vi "Write SPI.vi"(8 "error in (no error)":errorcluster, 10 "LINX SPI":refnum<class "LINX SPI.lvclass">, 11 "LINX-ADS1015 in":refnum<class "LINX-ADS1256.lvclass">) -> (0 "error out":errorcluster, 3 "LINX-ADS1015 out":refnum<class "LINX-ADS1256.lvclass">)   [LabVIEW 2020, in "LINX-ADS1256.lvclass"]
uses:
  LINX-ADS1256.lvclass
  LINX SPI/LINX SPI.lvclass
  LINX-ADS1256.lvclass/LINX-ADS1256.ctl
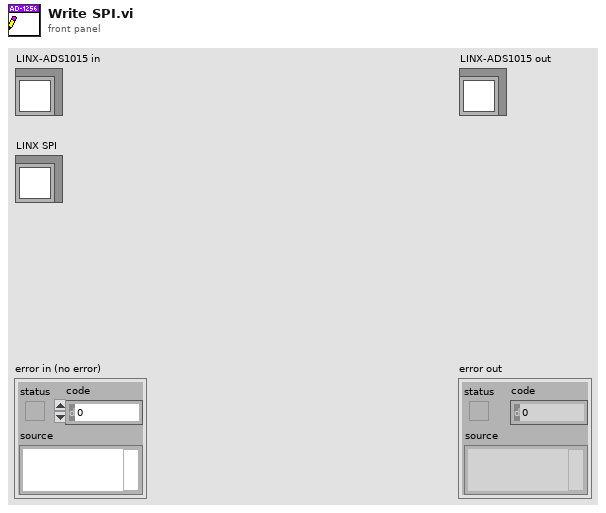
[diagram p1: front panel]
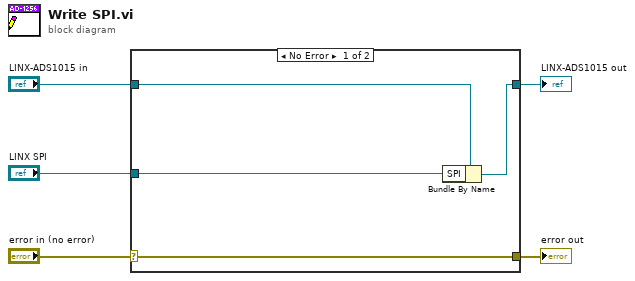
[diagram p0: block diagram]
diagram:
  n1 = case shown="No Error" "error in (no error)" {
    selector: "error in (no error)" -> [w9 w10]
    tunnel: [w9 w10] -> w4
    tunnel: [w7 w11] -> w2
    tunnel: "LINX-ADS1015 in" -> [w8 w11]
    tunnel: "LINX SPI" -> [w6 _]
    frame No Error {
      n2 = Bundle By Name(cluster=w8, "SPI"=w6) -> (w7:refnum<class "LINX-ADS1256.lvclass">)
    }
    frame Error {
    }
  }
  "error out" <- w4
  "LINX-ADS1015 out" <- w2
